vi "(26) part 2 que.vi"() -> ()   [LabVIEW 2025]
panel:
  in  "number: 0 to 2":dbl
  in  "number: 0 to 1":dbl
  in  "stop":bool
  out "x/y":dbl
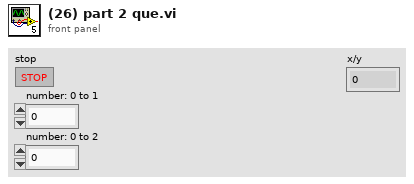
[diagram p1: front panel]
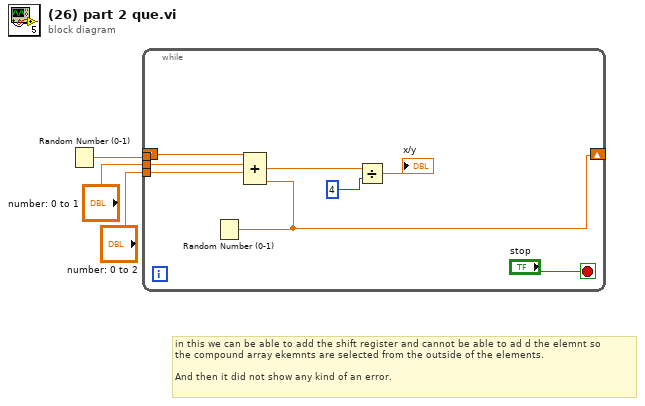
[diagram p0: block diagram]
diagram:
  # "in this we can be able to add the shift register and cannot be able to ad d the elemnt so \nthe compound array ekemnts are selected from the outside of the elements.\n\nAnd then it did not show any kind of an error."
  n1 = Random Number (0-1)() -> (number: 0 to 1=w3:dbl)
  n2 = while {
    shift-right: [w6] -> _
    shift-left: _ -> [w11]
    tunnel: w3 -> [_]
    tunnel: "number: 0 to 1" -> [w5]
    tunnel: "number: 0 to 2" -> [w4]
    stop <- "stop" stop-if-true
    n3 = Random Number (0-1)() -> (number: 0 to 1=w6:dbl)
    n4 = Compound Arithmetic op=ADD(w11, w5, w4, w6) -> (w10:dbl)
    n5 = Divide(x=w10, y=4) -> (x/y=→"x/y":dbl)
  }
